vi "System_Serial_Request.vi"(11 "input cluster":T1={"system"={"info"={"menuSelect"=0, "version"=0, "serial"="Test Sample", "captureActive"=FALSE, "captureBegin"=FALSE, "emptyAndRefill"=FALSE}, "userInfo"={"operatorName"="", "date"=timestamp(2713993200 s since 1904-01-01)}, "camera"={"exposureTime"=0, "aperture"=enum."Item 0", "framerate"=0, "framerateMax"=500, "legacyAttributes"=FALSE}}, "connections"={"arduino"={"connection"="", "status"=FALSE, "openState"=FALSE, "emptyStart"=0}, "pump"={"connection"="", "status"=FALSE, "command"="", "dispenseSpeed"=100, "flushSize"=100}, "camera"={"cam1"={"connection"="", "status"=FALSE}, "cam2"={"connection"="", "status"=FALSE}}}, "queue"={"process"={"cam1"=refnum, "cam2"=refnum, "queueSize"=0}, "save"={"cam1"=refnum, "cam2"=refnum, "queueSize"=0}, "overloadThreshold"=0}, "imageProcess"={"cam1"={"preAllocation"={"image"="Station", "originalDisplay"="Station", "originalRgb"="Station", "binary"="Station", "save"="Station", "calibrationFull"=refnum, "calibrationDetect"=refnum}, "calibration"={"pathFull"=path "C:/Users/au540322/Desktop/IHS_Project/images/Debris/Debris_0/Debris_0_2019_06_01-23-32-49-686.PNG", "pathDetect"=path "C:/Users/au540322/Desktop/IHS_Project/images/Debris/Debris_0/Debris_0_2019_06_01-23-32-49-686.PNG", "ROI"={"Left"=0, "Top"=0, "Right"=0, "Bottom"=0, "Rotation"=0.0}}}, "cam2"={"preAllocation"={"image"=refnum, "originalDisplay"=refnum, "originalRgb"=refnum, "binary"=refnum, "save"=refnum, "calibrationFull"=refnum, "calibrationDetect"=refnum}, "calibration"={"pathFull"=path "C:/Users/au540322/Desktop/IHS_Project/images/Debris/Debris_0/Debris_0_2019_06_01-23-32-49-686.PNG", "pathDetect"=path "C:/Users/au540322/Desktop/IHS_Project/images/Debris/Debris_0/Debris_0_2019_06_01-23-32-49-686.PNG", "ROI"={"Left"=0, "Top"=0, "Right"=0, "Bottom"=0, "Rotation"=0.0}}}, "process"={"planeExtract"=refnum, "planeSubtract"=refnum, "cropMask"=refnum}, "detection"={"sampleTimeout"=500, "sizeThreshold"=500, "detectionRegionPct"=0.0}}, "sampleData"={"sampleId"="", "projectId"="", "voucherID"="", "speciesName"="", "collectionDate"=timestamp(2713993200 s since 1904-01-01), "sampleStation"="", "location"="", "lat"=0.0, "lon"=0.0, "determiner"="", "sex"="", "otherNotes"=""}, "Session In"=""} {"sampleData"."collectionDate" format="%<%Y-%m-%d>T"; "imageProcess"."detection"."sizeThreshold" min=1; "imageProcess"."cam2"."calibration"."ROI"."Rotation" format="%.2f"; "imageProcess"."cam2"."calibration"."ROI"."Left" scale=0.0..1024.0; "imageProcess"."cam2"."calibration"."ROI"."Right" scale=0.0..1024.0; "imageProcess"."cam1"."calibration"."ROI"."Rotation" format="%.2f"; "imageProcess"."cam1"."calibration"."ROI"."Left" scale=0.0..1024.0; "imageProcess"."cam1"."calibration"."ROI"."Right" scale=0.0..1024.0; "queue"."overloadThreshold" min=1; "queue"."save"."queueSize" min=1; "queue"."process"."queueSize" min=1; "connections"."pump"."flushSize" min=1; "connections"."pump"."dispenseSpeed" min=1; "system"."camera"."framerateMax" min=1; "system"."userInfo"."date" format="%<%Y-%m-%dT%H:%M:%S+%z>T"; "system"."info"."version" items=["Standard", "XL"]; "system"."info"."menuSelect" items=["Session Data", "Extended Setup", "Buffer", "Camera", "Dispenser", "Stats", "Connections"]}) -> (3 "Output Cluster":T1={"system"={"info"={"menuSelect"=0, "version"=0, "serial"="Test Sample", "captureActive"=FALSE, "captureBegin"=FALSE, "emptyAndRefill"=FALSE}, "userInfo"={"operatorName"="", "date"=timestamp(2713993200 s since 1904-01-01)}, "camera"={"exposureTime"=0, "aperture"=enum."Item 0", "framerate"=0, "framerateMax"=500, "legacyAttributes"=FALSE}}, "connections"={"arduino"={"connection"="", "status"=FALSE, "openState"=FALSE, "emptyStart"=0}, "pump"={"connection"="", "status"=FALSE, "command"="", "dispenseSpeed"=100, "flushSize"=100}, "camera"={"cam1"={"connection"="", "status"=FALSE}, "cam2"={"connection"="", "status"=FALSE}}}, "queue"={"process"={"cam1"=refnum, "cam2"=refnum, "queueSize"=0}, "save"={"cam1"=refnum, "cam2"=refnum, "queueSize"=0}, "overloadThreshold"=0}, "imageProcess"={"cam1"={"preAllocation"={"image"="Station", "originalDisplay"="Station", "originalRgb"="Station", "binary"="Station", "save"="Station", "calibrationFull"=refnum, "calibrationDetect"=refnum}, "calibration"={"pathFull"=path "C:/Users/au540322/Desktop/IHS_Project/images/Debris/Debris_0/Debris_0_2019_06_01-23-32-49-686.PNG", "pathDetect"=path "C:/Users/au540322/Desktop/IHS_Project/images/Debris/Debris_0/Debris_0_2019_06_01-23-32-49-686.PNG", "ROI"={"Left"=0, "Top"=0, "Right"=0, "Bottom"=0, "Rotation"=0.0}}}, "cam2"={"preAllocation"={"image"=refnum, "originalDisplay"=refnum, "originalRgb"=refnum, "binary"=refnum, "save"=refnum, "calibrationFull"=refnum, "calibrationDetect"=refnum}, "calibration"={"pathFull"=path "C:/Users/au540322/Desktop/IHS_Project/images/Debris/Debris_0/Debris_0_2019_06_01-23-32-49-686.PNG", "pathDetect"=path "C:/Users/au540322/Desktop/IHS_Project/images/Debris/Debris_0/Debris_0_2019_06_01-23-32-49-686.PNG", "ROI"={"Left"=0, "Top"=0, "Right"=0, "Bottom"=0, "Rotation"=0.0}}}, "process"={"planeExtract"=refnum, "planeSubtract"=refnum, "cropMask"=refnum}, "detection"={"sampleTimeout"=500, "sizeThreshold"=500, "detectionRegionPct"=0.0}}, "sampleData"={"sampleId"="", "projectId"="", "voucherID"="", "speciesName"="", "collectionDate"=timestamp(2713993200 s since 1904-01-01), "sampleStation"="", "location"="", "lat"=0.0, "lon"=0.0, "determiner"="", "sex"="", "otherNotes"=""}, "Session In"=""} {"sampleData"."collectionDate" format="%<%Y-%m-%d>T"; "imageProcess"."detection"."sizeThreshold" min=1; "imageProcess"."cam2"."calibration"."ROI"."Rotation" format="%.2f"; "imageProcess"."cam2"."calibration"."ROI"."Left" scale=0.0..1024.0; "imageProcess"."cam2"."calibration"."ROI"."Right" scale=0.0..1024.0; "imageProcess"."cam1"."calibration"."ROI"."Rotation" format="%.2f"; "imageProcess"."cam1"."calibration"."ROI"."Left" scale=0.0..1024.0; "imageProcess"."cam1"."calibration"."ROI"."Right" scale=0.0..1024.0; "queue"."overloadThreshold" min=1; "queue"."save"."queueSize" min=1; "queue"."process"."queueSize" min=1; "connections"."pump"."flushSize" min=1; "connections"."pump"."dispenseSpeed" min=1; "system"."camera"."framerateMax" min=1; "system"."userInfo"."date" format="%<%Y-%m-%dT%H:%M:%S+%z>T"; "system"."info"."version" items=["Standard", "XL"]; "system"."info"."menuSelect" items=["Session Data", "Extended Setup", "Buffer", "Camera", "Dispenser", "Stats", "Connections"]}, 5 "read buffer":string)   [LabVIEW 2022 SP3]
uses:
  controls/Data.ctl
  <vilib>/userdefined/High Color/IMAQdx.ctl
  <vilib>/vision/Image Controls.llb/IMAQ Image.ctl
  bb14c998-3f04-4b67-919d-3d21de235356.vi
  <vilib>/regexp/Match Regular Expression.xnode
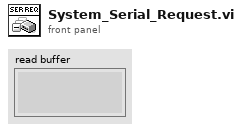
[diagram p1: front panel]
types:
  T1 = typedef "Data.ctl" = cluster{"system":cluster{"info":cluster{"menuSelect":u16, "version":u16, "serial":string, "captureActive":bool, "captureBegin":bool, "emptyAndRefill":bool}, "userInfo":cluster{"operatorName":string, "date":timestamp}, "camera":cluster{"exposureTime":i32, "aperture":enum32{"Item 0", "Item 1", "Item 2", "Item 3"}, "framerate":i32, "framerateMax":i32, "legacyAttributes":bool}}, "connections":cluster{"arduino":cluster{"connection":refnum<visa-resource-name>, "status":bool, "openState":bool, "emptyStart":u32}, "pump":cluster{"connection":refnum<visa-resource-name>, "status":bool, "command":string, "dispenseSpeed":i32, "flushSize":i32}, "camera":cluster{"cam1":cluster{"connection":T2, "status":bool}, "cam2":cluster{"connection":T2, "status":bool}}}, "queue":cluster{"process":cluster{"cam1":refnum<queue>, "cam2":refnum<queue>, "queueSize":i32}, "save":cluster{"cam1":refnum<queue>, "cam2":refnum<queue>, "queueSize":i32}, "overloadThreshold":i32}, "imageProcess":cluster{"cam1":cluster{"preAllocation":cluster{"image":T3, "originalDisplay":T3, "originalRgb":T3, "binary":T3, "save":T3, "calibrationFull":T3, "calibrationDetect":T3}, "calibration":cluster{"pathFull":path, "pathDetect":path, "ROI":T4}}, "cam2":cluster{"preAllocation":cluster{"image":T3, "originalDisplay":T3, "originalRgb":T3, "binary":T3, "save":T3, "calibrationFull":T3, "calibrationDetect":T3}, "calibration":cluster{"pathFull":path, "pathDetect":path, "ROI":T4}}, "process":cluster{"planeExtract":T3, "planeSubtract":T3, "cropMask":T3}, "detection":cluster{"sampleTimeout":i32, "sizeThreshold":i32, "detectionRegionPct":dbl}}, "sampleData":cluster{"sampleId":string, "projectId":string, "voucherID":string, "speciesName":string, "collectionDate":timestamp, "sampleStation":string, "location":string, "lat":dbl, "lon":dbl, "determiner":string, "sex":string, "otherNotes":string}, "Session In":T2}
  T2 = typedef "IMAQdx.ctl" = refnum<k21>
  T3 = typedef "IMAQ Image.ctl" = refnum<image>
  T4 = typedef "IMAQ Rectangle" = cluster{"Left":i32, "Top":i32, "Right":i32, "Bottom":i32, "Rotation":dbl}
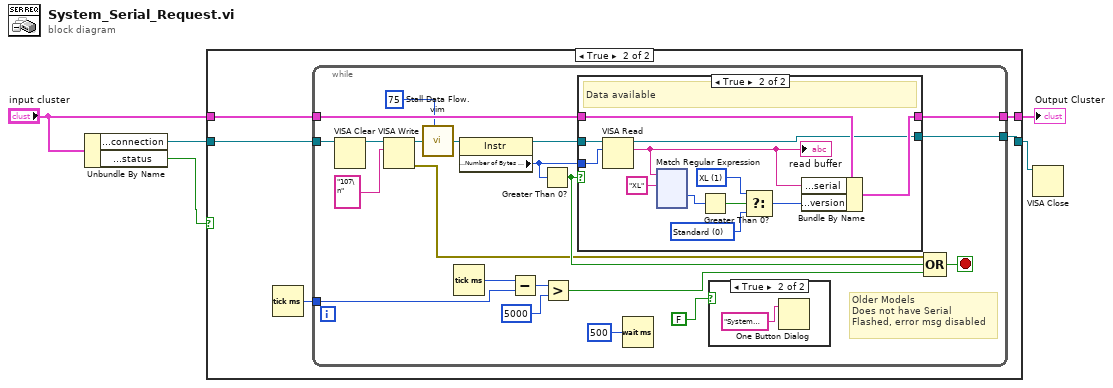
[diagram p0: block diagram]
diagram:
  n1 = Unbundle By Name("input cluster") -> ("connections.arduino.connection"=w1:refnum<visa-resource-name>, "connections.arduino.status"=w2:bool)
  n2 = case shown="True" w2 {
    tunnel: w1 -> [w6 w9]
    tunnel: "input cluster" -> [w7 w11]
    tunnel: [w7 w10] -> w4
    tunnel: [w6 w8] -> w3
    frame False {
    }
    frame True {
      n3 = Tick Count (ms)() -> (millisecond timer value=w12:u32)
      n4 = while {
        tunnel: w12 -> [w25]
        tunnel: w11 -> [w23]
        tunnel: [w22] -> w10
        tunnel: w9 -> [w17]
        tunnel: [w19] -> w8
        stop <- w30 stop-if-true
        # "Older Models\nDoes not have Serial\nFlashed, error msg disabled"
        n5 = VISA Clear(VISA resource name=w17) -> (VISA resource name out=w16:refnum<visa-resource-name>)  [unwired: 1 in, 1 out]
        n6 = VISA Write(VISA resource name=w16, write buffer="107\n") -> (VISA resource name out=w20:refnum<visa-resource-name>, error out=w21:errorcluster)  [unwired: 1 in, 1 out]
        n7 = call "Stall Data Flow.vim"("value in"=w20, "milliseconds to wait"=u32 75) -> ("value out"=w15:refnum<visa-resource-name>)  [unwired: 1 out]
        n8 = Tick Count (ms)() -> (millisecond timer value=w27:u32)
        n9 = property class="Instr"(reference=w15) -> (reference out=w32:refnum<visa-resource-name>, "Serial Settings:Number of Bytes at Serial Port"=w33:u32)  [unwired: 1 in, 1 out]
        n10 = Subtract(x=w27, y=w25) -> (x-y=w28:u32)
        n11 = Greater Than 0?(x=w33) -> (x > 0?=w29:bool)
        n12 = Greater?(x=w28, y=u32 5000 ("x")) -> (0:w24:bool)
        n13 = case shown="True" w29 {
          tunnel: w33 -> [_ w47]
          tunnel: w32 -> [w34 w46]
          tunnel: w23 -> [w35 w43]
          tunnel: [w35 w42] -> w22
          tunnel: [w34 w36] -> w19
          frame False {
            # "No data"
          }
          frame True {
            w39 = u16 1 items=["Standard", "XL"] ("SystemVersion")
            w40 = u16 0 items=["Standard", "XL"] ("SystemVersion")
            # "Data available"
            n14 = VISA Read(VISA resource name=w46, byte count=w47) -> (VISA resource name out=w36:refnum<visa-resource-name>, read buffer=w37:string)  [unwired: 1 in, 2 out]
            "read buffer" <- w37
            n15 = xnode "Match Regular Expression"("input string"=w37, "regular expression"="XL") -> ("offset past match"=w44:i32)  [unwired: 4 in, 4 out]
            n16 = Greater Than 0?(x=w44) -> (x > 0?=w41:bool)
            n17 = Select(t=w39, s=w41, f=w40) -> (s? t:f=w38:u16)
            n18 = Bundle By Name(cluster=w43, "system.info.serial"=w37, "system.info.version"=w38) -> (w42:T1)
          }
        }
        n19 = Wait (ms)(milliseconds to wait=u32 500) -> ()  [unwired: 1 out]
        n20 = case shown="True" FALSE {
          frame False {
          }
          frame True {
            n21 = One Button Dialog(message="System Serial Request Error!\nCommunication timed out") -> ()  [unwired: 1 in, 1 out]
          }
        }
        n22 = Compound Arithmetic op=OR(w21, w29, w24) -> (w30:bool)
      }
    }
  }
  "Output Cluster" <- w4
  n23 = VISA Close(VISA resource name=w3) -> ()  [unwired: 1 in, 1 out]
